vi "TCam_HorizontalLines.vi"(7 "Width":u32, 8 "error in (no error)":errorcluster, 9 "Cluster":T1 {"Points"."Top Left"."Y" format="%.2f"; "Points"."Top Left"."X" format="%.2f"; "Points"."Top Right"."Y" format="%.2f"; "Points"."Top Right"."X" format="%.2f"; "Points"."Bottom Left"."Y" format="%.2f"; "Points"."Bottom Left"."X" format="%.2f"; "Points"."Bottom Right"."Y" format="%.2f"; "Points"."Bottom Right"."X" format="%.2f"; "Points"."Fixpoint"."Y" format="%.2f"; "Points"."Fixpoint"."X" format="%.2f"}, 10 "Size":u16, 11 "Refnum in":T2) -> (0 "error out":errorcluster, 3 "Refnum out":T2)   [LabVIEW 2020]
uses:
  <vilib>/vision/Image Controls.llb/IMAQ Image.ctl
  DataCluster_TCAL.ctl
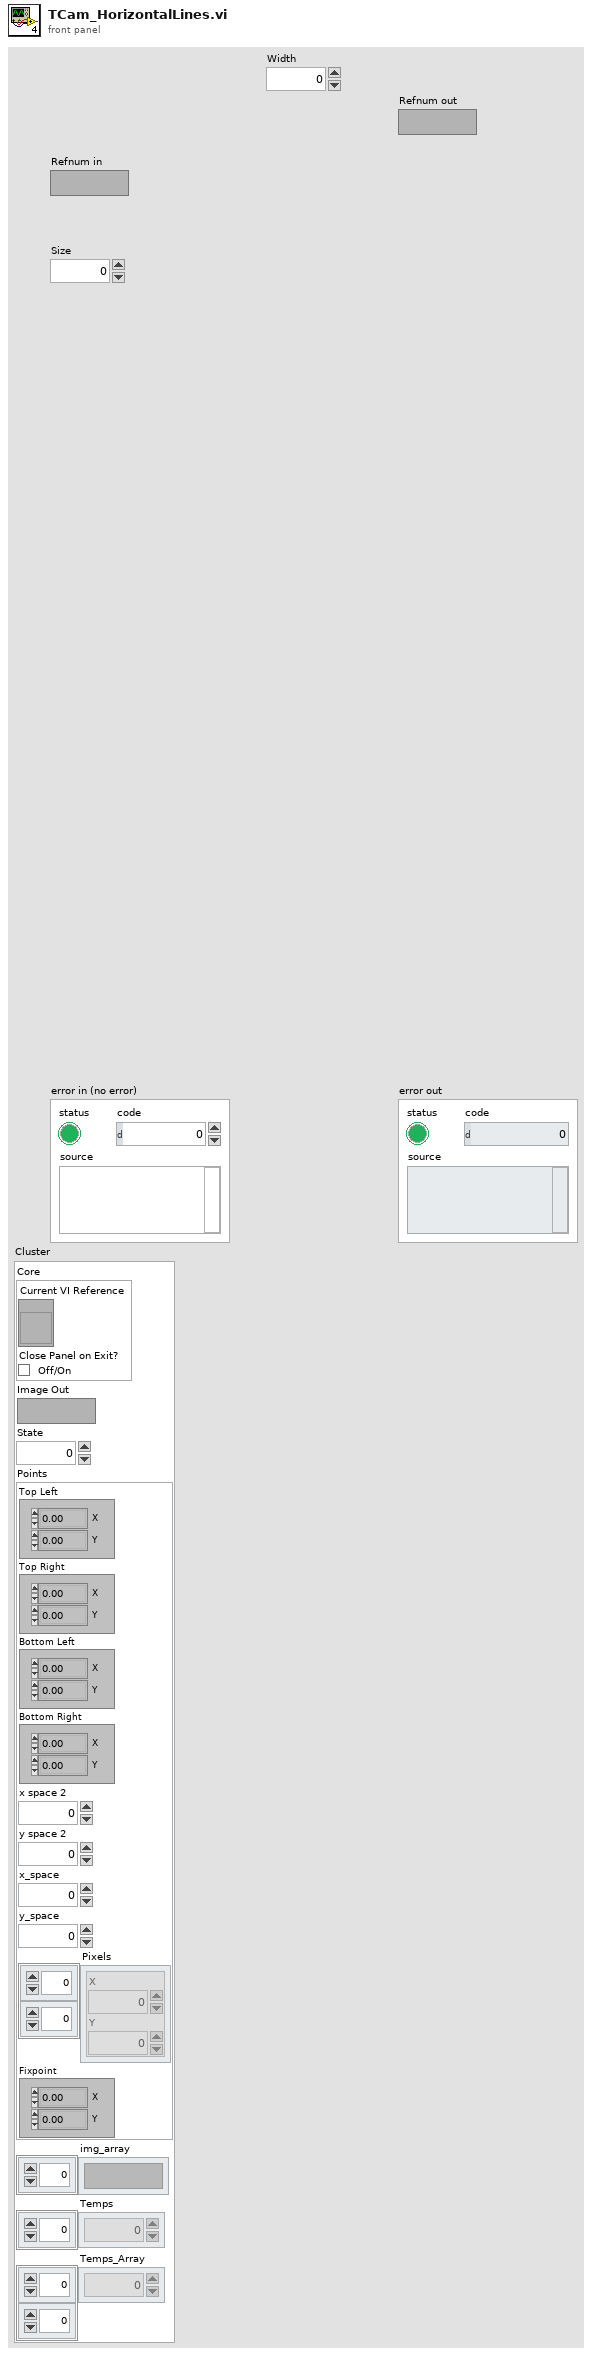
[diagram p1: front panel]
types:
  T1 = typedef "DataCluster_TCAL.ctl" = cluster{"Core":cluster{"Current VI Reference":refnum<vi>, "Close Panel on Exit?":bool}, "Image Out":T2, "State":i32, "Points":cluster{"Top Left":T3, "Top Right":T3, "Bottom Left":T3, "Bottom Right":T3, "x space 2":dbl, "y space 2":sgl, "x_space":sgl, "y_space":sgl, "Pixels":cluster{"X":i32, "Y":i32}[][], "Fixpoint":T3}, "img_array":T2[], "Temps":dbl[], "Temps_Array":dbl[][]}
  T2 = typedef "IMAQ Image.ctl" = refnum<image>
  T3 = typedef "IMAQ Point" = cluster{"X":sgl, "Y":sgl}
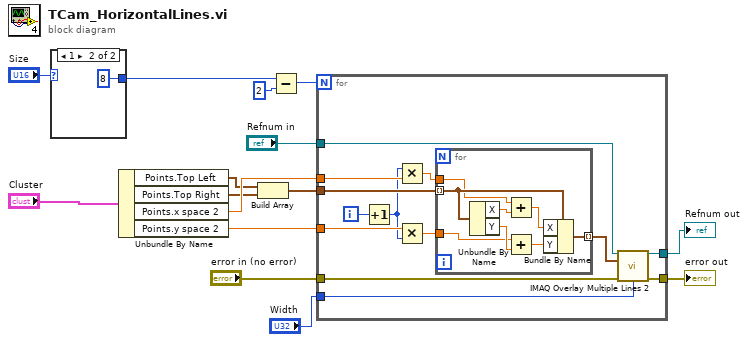
[diagram p0: block diagram]
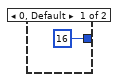
[diagram p2: hidden frame]
diagram:
  n1 = case shown="1" "Size" {
    tunnel: [16 8] -> w15
    frame 0, Default {
    }
    frame 1 {
    }
  }
  n2 = Unbundle By Name("Cluster") -> ("Points.Top Left"=w7:T3, "Points.Top Right"=w8:T3, "Points.x space 2"=w11:dbl, "Points.y space 2"=w10:sgl)
  n3 = Build Array(w7, w8) -> (w9:T3[])
  n4 = Subtract(x=w15, y=u16 2) -> (x-y=w12:i32)
  n5 = for {
    N: w12 -> [_]
    tunnel: "Refnum in" -> [w30]
    tunnel: [w29] -> w3
    tunnel: "error in (no error)" -> [w28]
    tunnel: [w27] -> w5
    tunnel: "Width" -> [w26]
    tunnel: w9 -> [w25]
    tunnel: w10 -> [w24]
    tunnel: w11 -> [w23]
    i -> [w20]
    n6 = Increment(x=w20) -> (x+1=w18:i32)
    n7 = Multiply(x=w18, y=w23) -> (x*y=w19:dbl)
    n8 = Multiply(x=w24, y=w18) -> (x*y=w21:sgl)
    n9 = for {
      tunnel: w25 -> [w38] mode=indexing
      tunnel: w21 -> [w33]
      tunnel: w19 -> [w32]
      tunnel: [w31] -> w22 mode=indexing
      n10 = Unbundle By Name(w38) -> ("X"=w37:sgl, "Y"=w35:sgl)
      n11 = Add(x=w32, y=w37) -> (x+y=w36:dbl)
      n12 = Add(x=w33, y=w35) -> (x+y=w34:sgl)
      n13 = Bundle By Name(cluster=w38, "X"=w36, "Y"=w34) -> (w31:T3)
    }
    n14 = call "IMAQ Overlay Multiple Lines 2"("Image"=w30, "Line End Points"=w22, "error in (no error)"=w28, "Width"=w26) -> ("Image Out"=w29:T2, "error out"=w27:errorcluster)  [unwired: 10 in]
  }
  "error out" <- w5
  "Refnum out" <- w3
